vi "Read Header.vi"(8 "error in":errorcluster, 11 "SLL in":refnum<class "SLL.lvclass">) -> (0 "error out":errorcluster, 2 "Header":string[](array[string]), 3 "SLL out":refnum<class "SLL.lvclass">)   [LabVIEW 2023, in "SLL.lvlib" / "SLL.lvclass"]
uses:
  SLL.lvclass
  SLL.lvclass/SLL.ctl
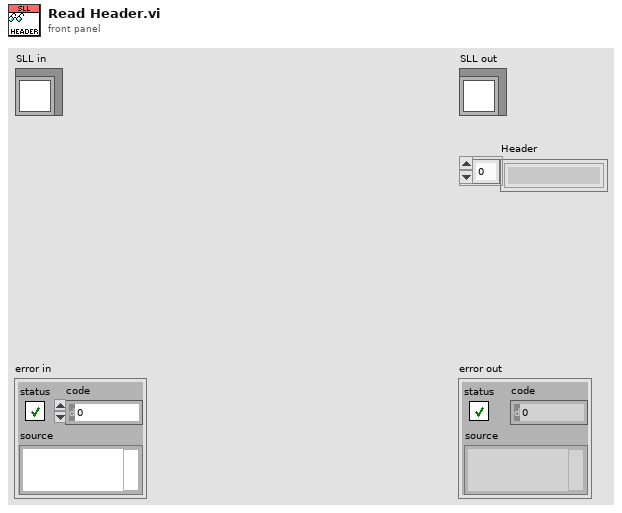
[diagram p1: front panel]
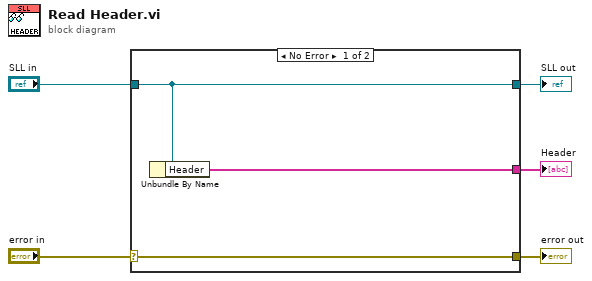
[diagram p0: block diagram]
diagram:
  n1 = case shown="No Error" "error in" {
    selector: "error in" -> [w8 w9]
    tunnel: [w8 w9] -> w4
    tunnel: [w7 w10] -> w2
    tunnel: "SLL in" -> [w7 w10]
    tunnel: [w6 _] -> w1
    frame No Error {
      n2 = Unbundle By Name(w7) -> ("Header"=w6:string[])
    }
    frame Error {
    }
  }
  "error out" <- w4
  "SLL out" <- w2
  "Header" <- w1
